vi "Get Public API.vi"(8 "error in (no error)":errorcluster, 11 "instrument.Cryostation in":refnum<class "instrument.Cryostation.lvclass">) -> (0 "error out":errorcluster, 2 "Commands":string[](array[string]), 3 "instrument.Cryostation out":refnum<class "instrument.Cryostation.lvclass">)   [LabVIEW 2016, in "instrument.Cryostation.lvclass"]
uses:
  instrument.Cryostation.lvclass
  Typedefs/Commands-enum.ctl
  <userlib>/LevyLab/Levylab Instruments/Instrument Types/Cryostat/Instrument.Cryostat.lvclass
panel:
  in  "Enum":T1
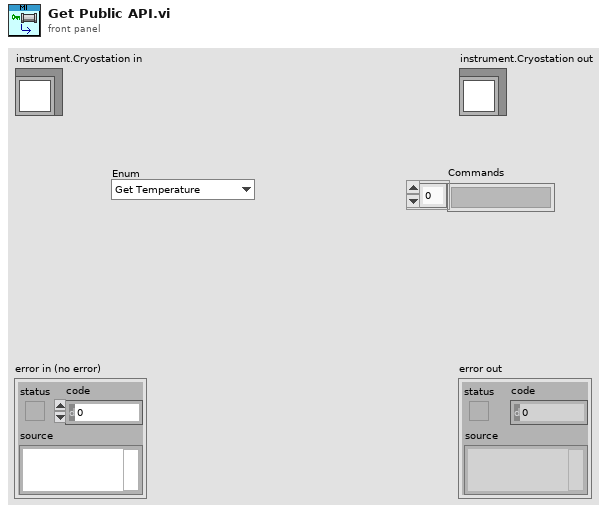
[diagram p1: front panel]
types:
  T1 = typedef "instrument.Cryostation.lvclass/Commands-enum.ctl" = enum16{"Get Temperature", "getAll"}
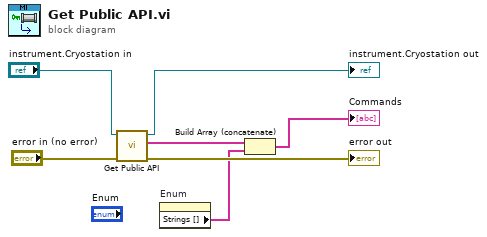
[diagram p0: block diagram]
diagram:
  n1 = call-parent "Get Public API.vi"("error in (no error)"="error in (no error)", "Instrument in"="instrument.Cryostation in") -> ("error out"=→"error out":errorcluster, "Commands"=w2:string[], "Instrument out"=→"instrument.Cryostation out":refnum<class "instrument.Cryostation.lvclass">)  [unwired: 7 in]
  n2 = property on="Enum" class="Enum (strict)"() -> ("Strings []"=w1:string[])  [unwired: 2 in, 2 out]
  n3 = Build Array (concatenate)(w2, w1) -> (→"Commands":string[])
